vi "Multiple Connections - Client 1.vi"() -> ()   [LabVIEW 2016]
doc: "Establishes a connection to the specified host and port and reads the date and time data sent by the Server. It first reads 4 bytes defining the length of the date & time string and then reads the data. After you click the stop button, this VI sends a single character to tell the Date Server VI to terminate the connection.\n\n<B>Note:</B> Requires the use of the Multiple Connections - Server.vi."
panel:
  in  "stop":bool
  out "Date - Time":string
  in  "Machine":string="localhost"
  in  "Port":u16=6341
  # "Instructions:\n1. Open the Multiple Connections - Server.vi.\n2. Run the Multiple Connections - Server.vi first.\n3. Run the Client VIs second.\n4. Stop this VI and restart it to notice the # of Connections on the Server VI change.\n5. Stop the Server VI.  This VI will stop when it times out."
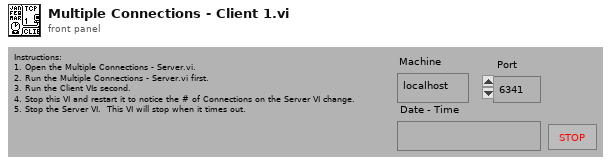
[diagram p1: front panel]
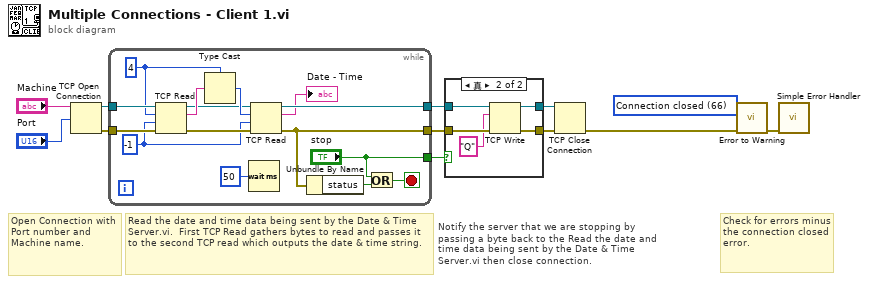
[diagram p0: block diagram]
diagram:
  w1 = 66 items=["No Error", "Argument Error", "Memory Full", "Out of Zone", "End of File", "File Already Open", "Generic File IO Error", "File Not Found", "File Permission Error", "Disk Full", "Duplicate Path", "Too Many Files Open", "Not Enabled", "Resource File Not Found", "Cannot Add Resource", "Resource Not Found", "Image Not Found", "Image Memory Error", "Pen Does Not Exist", "Config Bad Type", "Config Token Not Found", "Config Parse Error", "Config Memory Error", "Bad External Code Format", "Bad External Code Offset", "External Code Not Present", "Null Window", "Destroy Window Mixup", "Null Menu", "Print Aborted", "Bad Print Record", "Print Driver Error", "Windows Error During Print", "Memory Error During Print", "Print Dialog Error", "Generic Print Error", "Invalid Device Refnum", "Device Not Found", "Device Parameter Error", "Device Unit Error", "Can't Open Device", "Device Call Aborted", "Generic Error", "Cancelled By User", "Object ID Too Low", "Object ID Too High", "Object Not In Heap", "Unknown Heap", "Bad DefProc ID", "DefProc Not In Table", "Message Out Of Range", "Null Method", "Unknown Message", "Manager Call Not Supported", "Bad address", "Connection In progress", "Connection timed out", "Connection is already in progress", "Network attribute not supported", "Network error", "Address in use", "System out of memory", "Connection aborted", "Connection refused", "Connection is not connected", "Connection is already connected", "Connection closed", "Initialize error (interapplication manager)", "Bad occurrence", "Wait on unbound occurrence handler", "Occurrence queue overflow", "Bad path", "Semaphore not signaled", "Unrecognized type (interapplication manager)"] ("1st Error to Convert")
  # "Check for errors minus the connection closed error."
  # "Read the date and time data being sent by the Date & Time Server.vi.  First TCP Read gathers bytes to read and passes it to the second TCP read which outputs the date & time string."
  # "Open Connection with Port number and Machine name."
  n1 = TCP Open Connection(address="Machine", remote port or service name="Port") -> (connection ID=w10:refnum<k5>, error out=w9:errorcluster)  [unwired: 1 in, 2 out]
  n2 = while {
    tunnel: ["stop"] -> w4
    tunnel: [w20] -> w8
    tunnel: [w16] -> w6
    tunnel: w9 -> [w26]
    tunnel: w10 -> [w27]
    stop <- w17 stop-if-true
    w19 = -1
    w25 = 4
    n3 = TCP Read(connection ID=w27, bytes to read=w25, error in (no error)=w26, 9:w19) -> (connection ID out=w21:refnum<k5>, data out=w24:string, error out=w23:errorcluster)  [unwired: 1 out]
    n4 = Type Cast(type=w25, x=w24) -> (*(type *) &x=w22:i32)
    n5 = Wait (ms)(milliseconds to wait=u32 50) -> ()  [unwired: 1 out]
    n6 = TCP Read(connection ID=w21, bytes to read=w22, error in (no error)=w23, 9:w19) -> (connection ID out=w20:refnum<k5>, data out=→"Date - Time":string, error out=w16:errorcluster)  [unwired: 1 out]
    n7 = Unbundle By Name(w16) -> ("status"=w15:bool)
    n8 = Or(x="stop", y=w15) -> (x .or. y?=w17:bool)
  }
  n9 = case "Notify the server that we are stopping by passing a byte back to the Read the date and time data being sent by the Date & Time Server.vi then close connection." shown="真" w4 {
    tunnel: w8 -> [w29 w34]
    tunnel: [w29 w32] -> w7
    tunnel: w6 -> [w28 w33]
    tunnel: [w28 w31] -> w5
    frame False {
    }
    frame True {
      n10 = TCP Write(connection ID=w34, data in="Q", error in (no error)=w33) -> (connection ID out=w32:refnum<k5>, error out=w31:errorcluster)  [unwired: 2 out]
    }
  }
  n11 = TCP Close Connection(connection ID=w7, error in (no error)=w5) -> (error out=w3:errorcluster)  [unwired: 2 out]
  n12 = call <vilib>:"Error to Warning.vi"("1st Error to Convert"=w1, "error in"=w3) -> ("warning out"=w2:errorcluster)  [unwired: 3 in, 10 out]
  n13 = call <vilib>:"Simple Error Handler.vi"("error in (no error)"=w2) -> ()  [unwired: 1 in, 8 out]
